vi "Destroy Request Events.vi"(8 "error in":errorcluster) -> (0 "error out":errorcluster)   [LabVIEW 2020, in "Cycling by Event module.lvlib"]
doc: "Destroy the requests user events, even if there is an incoming error.\n\n<b>NOTE</b>: The contents of this VI are automatically generated and modified by the <b>Tools > DQMH Consortium > DQMH</b> utilities. Consider using those utilities instead of making your own modifications to this VI.\n_____\nBased on DQMH Project Template 7.0.1.1316."
uses:
  Cycling by Event module.lvlib
panel:
  # "NOTE: The contents of this VI are automatically generated and modified by the Tools > DQMH Consortium > DQMH utilities. Consider using those utilities instead of making your own modifications to this VI."
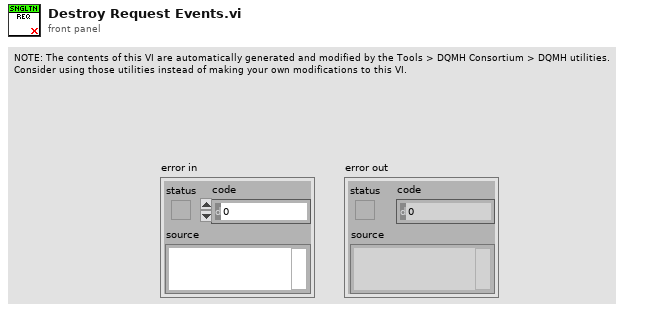
[diagram p1: front panel]
types:
  T1 = typedef "Cycling by Event module.lvlib/Request Events--cluster.ctl" = cluster{"Stop Module":refnum<user-event>, "Show Panel":refnum<user-event>, "Hide Panel":refnum<user-event>, "Get Module Execution Status":refnum<user-event>, "Show Diagram":refnum<user-event>, "Start cycling":refnum<user-event>, "Detecting 110rpm":refnum<user-event>, "Change state to HL":refnum<user-event>, "Detecting 100rpm":refnum<user-event>, "Detecting 0rpm":refnum<user-event>, "Stop cycling":refnum<user-event>}
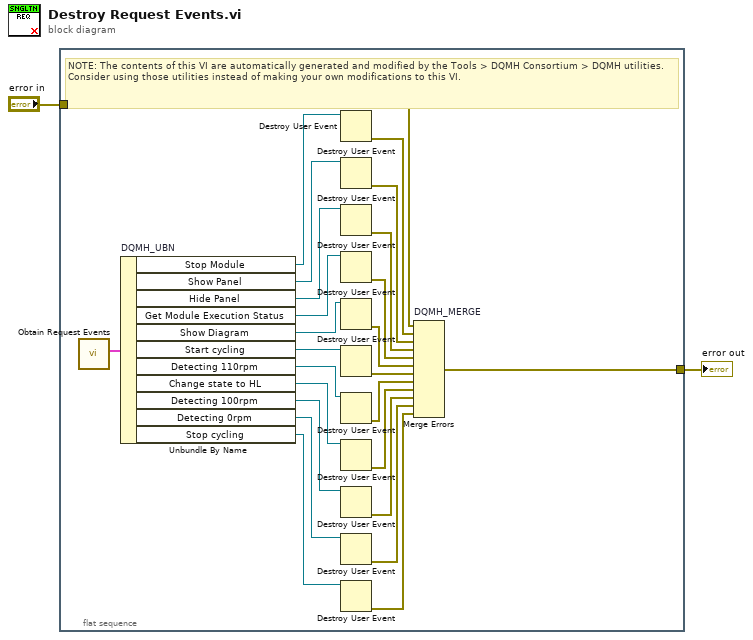
[diagram p0: block diagram]
diagram:
  n1 = flat-sequence {
    tunnel: [w26] -> w2
    tunnel: "error in" -> [w19]
    frame #0 {
      # "NOTE: The contents of this VI are automatically generated and modified by the Tools > DQMH Consortium > DQMH utilities. Consider using those utilities instead of making your own modifications to this VI."
      n2 = call "Obtain Request Events.vi"() -> ("Cycling by Event module Request Events"=w25:T1)  [unwired: 10 in, 1 out]
      n3 = Unbundle By Name "DQMH_UBN"(w25) -> ("Stop Module"=w24:refnum<user-event>, "Show Panel"=w21:refnum<user-event>, "Hide Panel"=w20:refnum<user-event>, "Get Module Execution Status"=w17:refnum<user-event>, "Show Diagram"=w15:refnum<user-event>, "Start cycling"=w13:refnum<user-event>, "Detecting 110rpm"=w11:refnum<user-event>, "Change state to HL"=w9:refnum<user-event>, "Detecting 100rpm"=w7:refnum<user-event>, "Detecting 0rpm"=w5:refnum<user-event>, "Stop cycling"=w3:refnum<user-event>)
      n4 = Destroy User Event(user event=w24) -> (error out=w27:errorcluster)  [unwired: 1 in]
      n5 = Destroy User Event(user event=w21) -> (error out=w23:errorcluster)  [unwired: 1 in]
      n6 = Destroy User Event(user event=w20) -> (error out=w22:errorcluster)  [unwired: 1 in]
      n7 = Destroy User Event(user event=w17) -> (error out=w18:errorcluster)  [unwired: 1 in]
      n8 = Destroy User Event(user event=w15) -> (error out=w16:errorcluster)  [unwired: 1 in]
      n9 = Destroy User Event(user event=w13) -> (error out=w14:errorcluster)  [unwired: 1 in]
      n10 = Destroy User Event(user event=w11) -> (error out=w12:errorcluster)  [unwired: 1 in]
      n11 = Destroy User Event(user event=w9) -> (error out=w10:errorcluster)  [unwired: 1 in]
      n12 = Destroy User Event(user event=w7) -> (error out=w8:errorcluster)  [unwired: 1 in]
      n13 = Destroy User Event(user event=w5) -> (error out=w6:errorcluster)  [unwired: 1 in]
      n14 = Destroy User Event(user event=w3) -> (error out=w4:errorcluster)  [unwired: 1 in]
      n15 = Merge Errors "DQMH_MERGE"(w19, w27, w23, w22, w18, w16, w14, w12, w10, w8, w6, w4) -> (w26:errorcluster)
    }
  }
  "error out" <- w2
